vi "createPolymorphicInstances.vi"(8 "error in (no error)":errorcluster, 10 "salTypdefPath":path=path "C:/LSSTSW/SAL_LabVIEW_Interface/SALTypedefs/Control 2.ctl", 11 "PolymorphicStructure in":refnum<class "PolymorphicStructure.lvclass">) -> (0 "error out":errorcluster, 3 "PolymorphicStructure out":refnum<class "PolymorphicStructure.lvclass">)   [LabVIEW 2012, in "PolymorphicStructure.lvclass"]
uses:
  PolymorphicStructure.lvclass
  OpenConnectionInstance/OpenConnectionInstance.lvclass
  WriteValueInstance/WriteValueInstance.lvclass
  ReadValueInstance/ReadValueInstance.lvclass
  CloseConnectionInstance/CloseConnectionInstance.lvclass
  PolymorphicStructure.lvclass/PolymorphicStructure.ctl
  PolymorphicInstance/PolymorphicInstance.lvclass
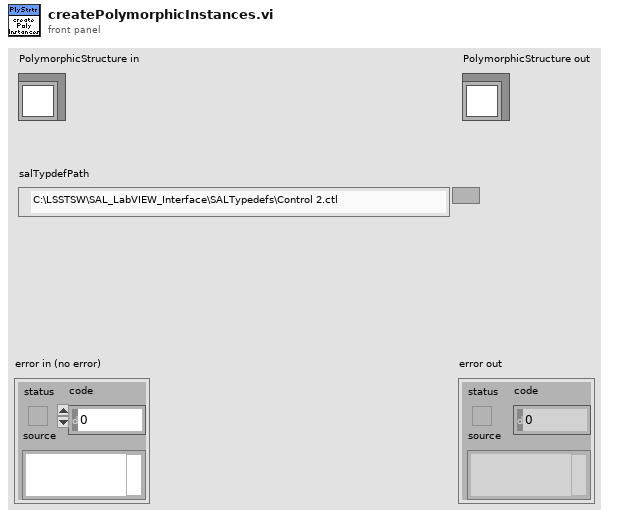
[diagram p1: front panel]
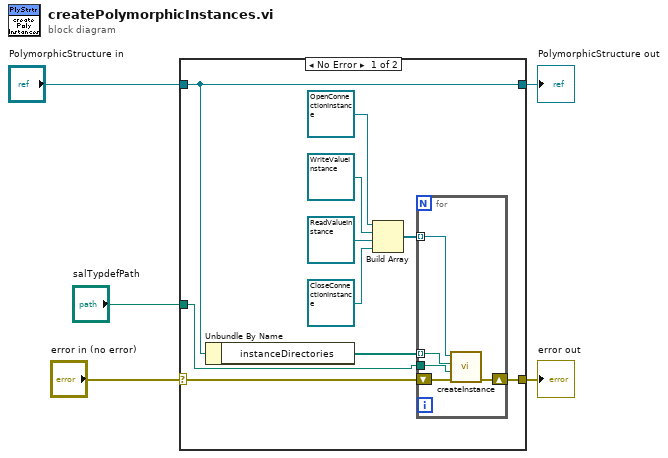
[diagram p0: block diagram]
diagram:
  n1 = case shown="No Error" "error in (no error)" {
    selector: "error in (no error)" -> [w7 w22]
    tunnel: [w6 w22] -> w4
    tunnel: [w15 w21] -> w2
    tunnel: "PolymorphicStructure in" -> [w15 w21]
    tunnel: "salTypdefPath" -> [w14 _]
    frame No Error {
      n2 = Unbundle By Name(w15) -> ("instanceDirectories"=w13:path[])
      n3 = Build Array(refnum<class "OpenConnectionInstance.lvclass"> refnum ("OpenConnectionInstance.lvclass"), refnum<class "WriteValueInstance.lvclass"> refnum ("WriteValueInstance.lvclass"), refnum<class "ReadValueInstance.lvclass"> refnum ("ReadValueInstance.lvclass"), refnum<class "CloseConnectionInstance.lvclass"> refnum ("CloseConnectionInstance.lvclass")) -> (w8:refnum<class "PolymorphicInstance.lvclass">[])
      n4 = for {
        tunnel: w14 -> [w20]
        tunnel: w13 -> [w19] mode=indexing
        tunnel: w8 -> [w18] mode=indexing
        shift-right: [w16] -> w6
        shift-left: w7 -> [w17]
        n5 = call-dynamic "createInstance.vi"("error in (no error)"=w17, "salTypedefPath"=w20, "instanceDirectory"=w19, "PolymorphicInstance in"=w18) -> ("error out"=w16:errorcluster)  [unwired: 6 in, 1 out]
      }
    }
    frame Error {
    }
  }
  "error out" <- w4
  "PolymorphicStructure out" <- w2
